vi "dummy data generator.vi"(11 "Size (128 kB)":u64(ring) items=["128 B"=128, "128 kB"=128000, "256 kB"=256000, "512 kB"=512000, "1 MB"=1000000, "1.2 MB"=1200000, "3 MB"=3000000, "8 MB"=8000000]) -> (2 "Array Size":i32, 3 "Byte Array":u8[](array[numeric]))   [LabVIEW 2020, in "Template.lvlib" / "Template.lvclass"]
doc: "Generates the desired byte array packet"
uses:
  Template.lvclass
  <vilib>/numeric/Random Number (Range) U64.vi
  <vilib>/numeric/sub_Random U32.vi
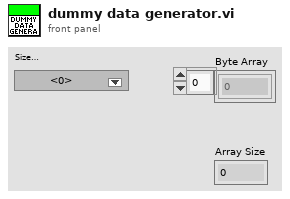
[diagram p1: front panel]
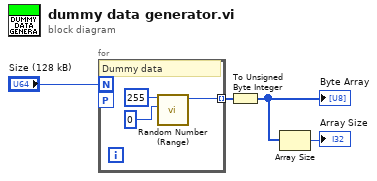
[diagram p0: block diagram]
diagram:
  n1 = for {
    N: "Size (128 kB)" -> [_]
    workers-P: _ -> [_]
    tunnel: [w5] -> w3 mode=indexing
    # "Dummy data"
    n2 = call-poly <vilib>:"Random Number (Range).vi"("lower bound (0)"=u64 0, "upper bound (100)"=u64 255) -> ("number"=w5:u64)  [unwired: 9 in]
  }
  n3 = To Unsigned Byte Integer(number=w3) -> (unsigned 8bit integer=w1:u8[])
  "Byte Array" <- w1
  n4 = Array Size(array=w1) -> (size(s)=→"Array Size":i32)
